vi "Configure.vi"(8 "error in (no error)":errorcluster, 9 "digital protocol settings":T1={"logic level"=enum."3.3 V", "PCM Data Configuration"={"Frame Sync Edge for Channel 0"=enum."Falling", "Channel Count Per Frame"=2, "Channel Length"=32, "Bit Depth"=24, "Channel 0 Offset"=1, "Endianness"=enum."MSB First", "Data Justification"=enum."Left Justified"}, "bit clock rate"=3025000.0, "master clock rate"=3025000.0, "clock mode"=enum."divided clock", "Frame Sync Clock Control"={"Frame Length"=64, "Frame Sync Pulse Width"=32, "Bit Clock Edge  Sync"=enum."Falling"}} {"master clock rate" format="%.4p"; "bit clock rate" format="%.4p"}, 10 "master clock channel list":string, 11 "data channel list":string) -> (0 "error out":errorcluster, 3 "digital serial task":refnum<class "Digital Serial.lvclass">)   [LabVIEW 2023, in "Digital Serial.lvclass"]
uses:
  Digital Serial.lvclass
  service/generation/controls/digital protocol settings.ctl
  <vilib>/PDM Acquisition Toolkit/host/Classes/Session/Controls/Logic Levels.ctl
  <vilib>/PDM Acquisition Toolkit/shared/controls/PCM Data Format Configuration.ctl
  <vilib>/PDM Acquisition Toolkit/shared/controls/Digital Edge.ctl
  <vilib>/PDM Acquisition Toolkit/shared/controls/PCM Bit Endianness.ctl
  <vilib>/PDM Acquisition Toolkit/shared/controls/PCM Data Justification.ctl
  <vilib>/PDM Acquisition Toolkit/shared/controls/clock mode.ctl
  <vilib>/PDM Acquisition Toolkit/shared/controls/PCM Frame Sync Control.ctl
  Digital Serial.lvclass/Digital Serial.ctl
  <vilib>/PDM Acquisition Toolkit/host/API/PDM Acquisition Toolkit.lvlib
  <vilib>/PDM Acquisition Toolkit/shared/PDM Shared.lvlib
  service/generation/controls/AudioGenTypeDefs.lvlib
  <vilib>/PDM Acquisition Toolkit/host/Classes/Session/DecoderSession.lvclass
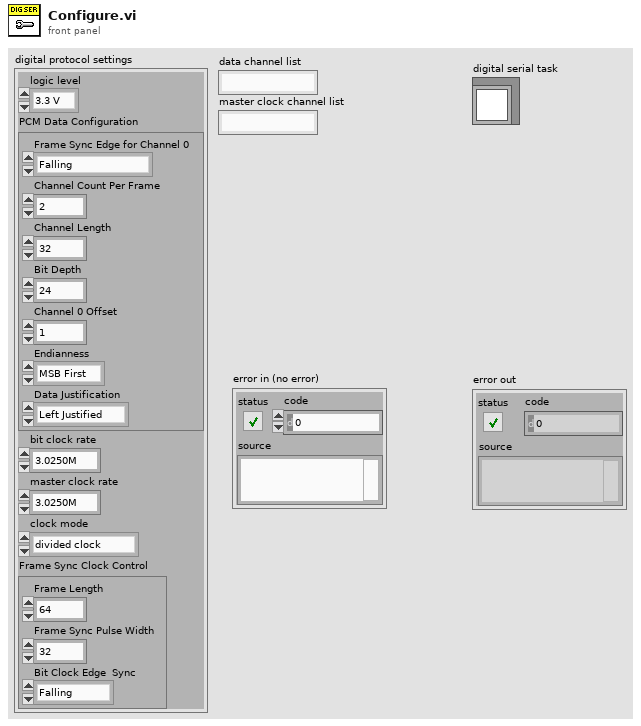
[diagram p1: front panel]
types:
  T1 = typedef "AudioGenTypeDefs.lvlib/digital protocol settings.ctl" = cluster{"logic level":T2, "PCM Data Configuration":T3, "bit clock rate":sgl, "master clock rate":sgl, "clock mode":T7, "Frame Sync Clock Control":T8}
  T2 = typedef "PDM Acquisition Class Library.lvlib/DecoderSession.lvclass/Logic Levels.ctl" = enum16{"3.3 V", "1.8 V", "1.2 V"}
  T3 = typedef "PDM Shared.lvlib/PCM Data Format Configuration.ctl" = cluster{"Frame Sync Edge for Channel 0":T4, "Channel Count Per Frame":u8, "Channel Length":u16, "Bit Depth":u8, "Channel 0 Offset":u16, "Endianness":T5, "Data Justification":T6}
  T4 = typedef "PDM Shared.lvlib/Digital Edge.ctl" = enum8{"Rising", "Falling"}
  T5 = typedef "PDM Shared.lvlib/PCM Bit Endianness.ctl" = enum16{"MSB First", "LSB First"}
  T6 = typedef "PDM Shared.lvlib/PCM Data Justification.ctl" = enum16{"Left Justified", "Right Justified"}
  T7 = typedef "PDM Shared.lvlib/clock mode.ctl" = enum16{"divided clock", "DDS"}
  T8 = typedef "PDM Shared.lvlib/PCM Frame Sync Control.ctl" = cluster{"Frame Length":u16, "Frame Sync Pulse Width":u16, "Bit Clock Edge  Sync":T4}
  T9 = typedef "PDM Acquisition Class Library.lvlib/PCM Output Task.lvclass/PCM Output Task DVR.ctl" = refnum<data-value>
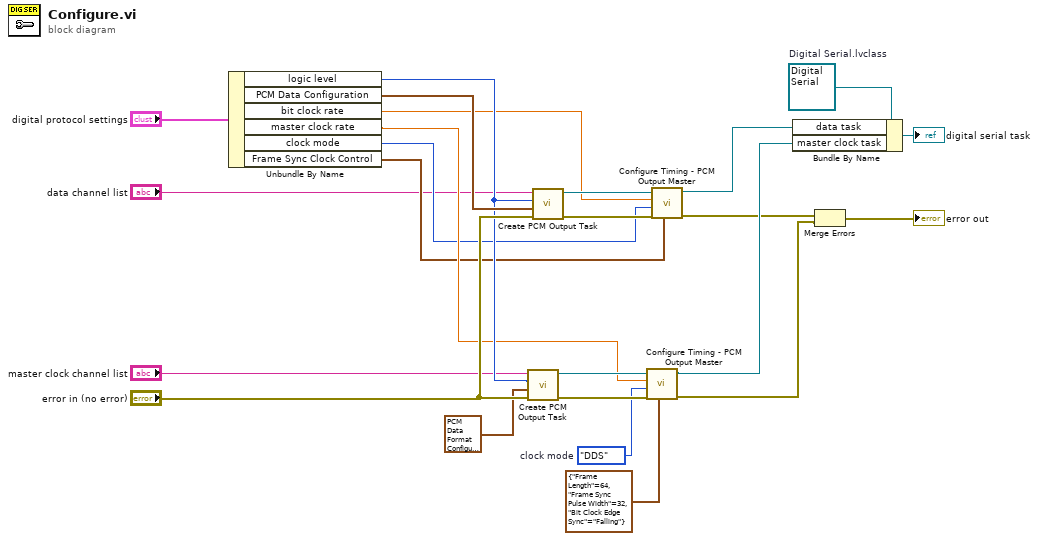
[diagram p0: block diagram]
diagram:
  w9 = refnum<class "Digital Serial.lvclass"> refnum  # Digital Serial.lvclass
  w20 = clock_mode."DDS"  # clock mode
  n1 = Unbundle By Name("digital protocol settings") -> ("logic level"=w14:T2, "PCM Data Configuration"=w16:T3, "bit clock rate"=w13:sgl, "master clock rate"=w12:sgl, "clock mode"=w11:T7, "Frame Sync Clock Control"=w10:T8)
  n2 = call <vilib>:"Create PCM Output Task.vi"("error in"="error in (no error)", "PCM data configuration"=T3 {"Frame Sync Edge for Channel 0"=enum."Falling", "Channel Count Per Frame"=2, "Channel Length"=32, "Bit Depth"=24, "Channel 0 Offset"=1, "Endianness"=enum."MSB First", "Data Justification"=enum."Left Justified"} ("PCM Data Configuration 2"), "logic level"=w14, "channel list"="master clock channel list") -> ("error out"=w21:errorcluster, "PCM output task out"=w22:T9)  [unwired: 6 in]
  n3 = call <vilib>:"Create PCM Output Task.vi"("error in"="error in (no error)", "PCM data configuration"=w16, "logic level"=w14, "channel list"="data channel list") -> ("error out"=w23:errorcluster, "PCM output task out"=w24:T9)  [unwired: 6 in]
  n4 = call <vilib>:"Configure Timing - PCM Output Master.vi"("Frame Sync Clock Control"=T8 {"Frame Length"=64, "Frame Sync Pulse Width"=32, "Bit Clock Edge  Sync"=enum."Falling"} ("Frame Sync Clock Control 2"), "error in"=w21, "clock mode"=w20, "Bit Clock rate"=w12, "PCM output task in"=w22) -> ("error out"=w2:errorcluster, "PCM output task out"=w3:T9)  [unwired: 4 in, 1 out]
  n5 = call <vilib>:"Configure Timing - PCM Output Master.vi"("Frame Sync Clock Control"=w10, "error in"=w23, "clock mode"=w11, "Bit Clock rate"=w13, "PCM output task in"=w24) -> ("error out"=w1:errorcluster, "PCM output task out"=w4:T9)  [unwired: 4 in, 1 out]
  n6 = Bundle By Name(cluster=w9, "data task"=w4, "master clock task"=w3) -> (→"digital serial task":refnum<class "Digital Serial.lvclass">)
  n7 = Merge Errors(w1, w2) -> (→"error out":errorcluster)
